vi "Client.vi"() -> ()   [LabVIEW 2020]
panel:
  in  "zone 6":bool
  in  "zone 5":bool
  in  "zone 4":bool
  in  "zone 3":bool
  in  "zone 2":bool
  in  "zone 1":bool
  in  "Alarm 6":bool
  in  "Alarm 5":bool
  in  "Alarm 4":bool
  in  "Alarm 3":bool
  in  "Alarm 2":bool
  in  "Alarm 1":bool
  in  "Bypass 6":bool
  in  "Bypass 5":bool
  in  "Bypass 4":bool
  in  "Bypass 3":bool
  in  "Bypass 2":bool
  in  "Bypass 1":bool
  in  "Temper 6":bool
  in  "Temper 5":bool
  in  "Temper 4":bool
  in  "Temper 3":bool
  in  "Temper 2":bool
  in  "Temper 1":bool
  # "1\n\n\n2\n\n\n3\n\n\n4\n\n\n5\n\n\n6"
  # "Bypass\nSwitches"
  # "Tamper\nSwitches"
  # "Alarm\nSwitches"
  # "Zone"
  # "Green = Normal\nRed = Alarm\nBlue = Bypass\nOrange = Tamper"
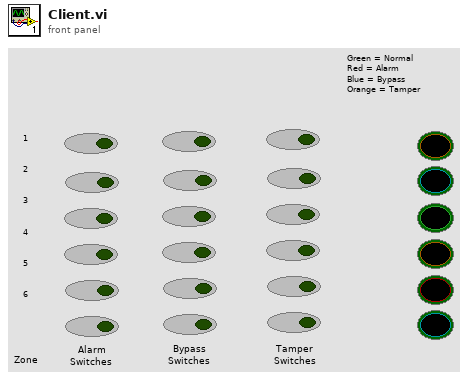
[diagram p1: front panel]
types:
  T1 = enum16{"Inti", "Wait", "zone 1", "zone 2", "zone 3", "zone 4", "zone 5", "zone 6"}
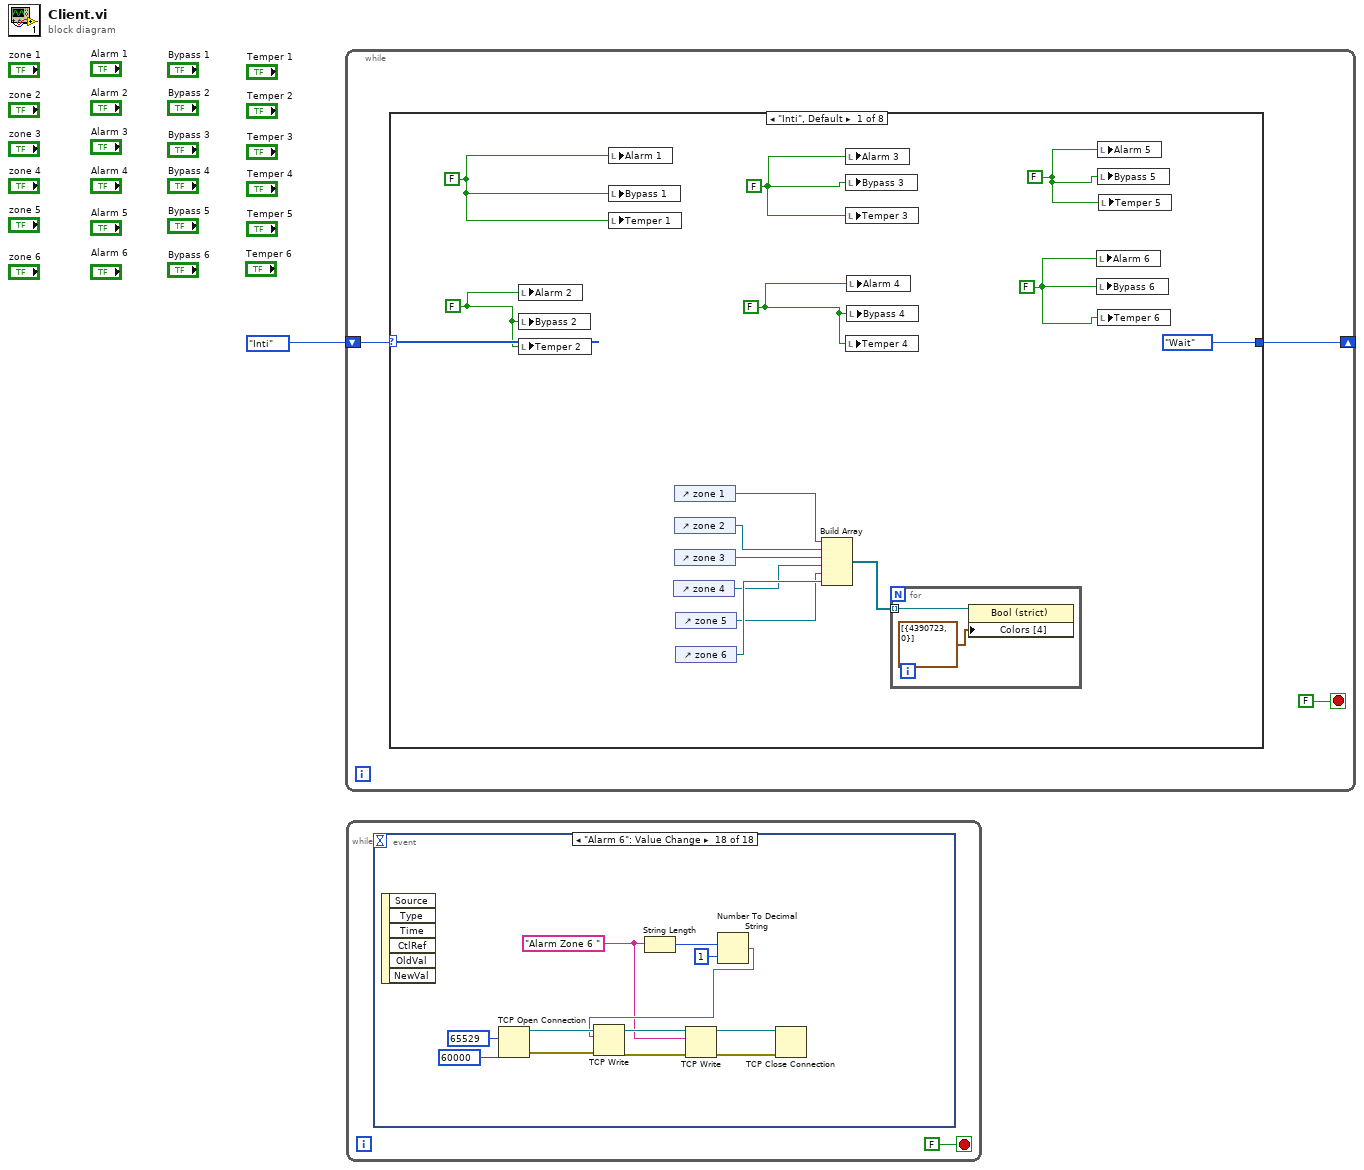
[diagram p0: block diagram]
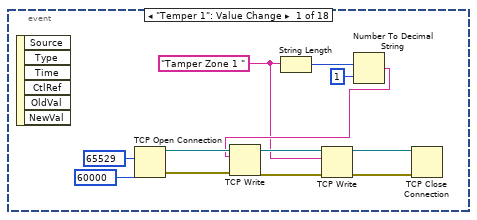
[diagram p2: hidden frame]
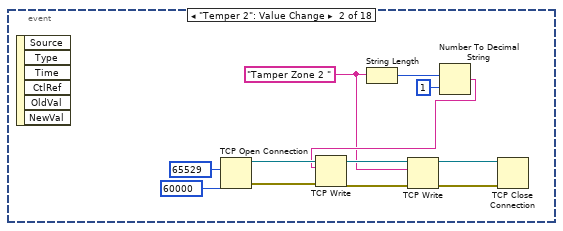
[diagram p3: hidden frame]
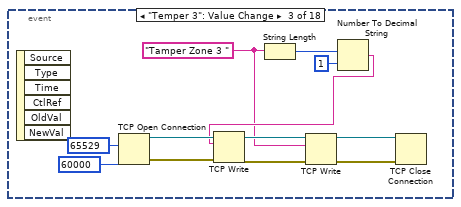
[diagram p4: hidden frame]
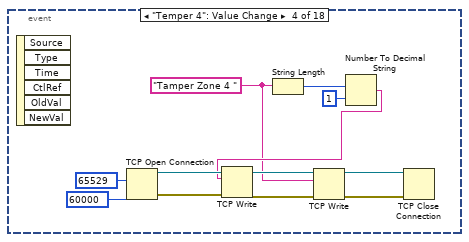
[diagram p5: hidden frame]
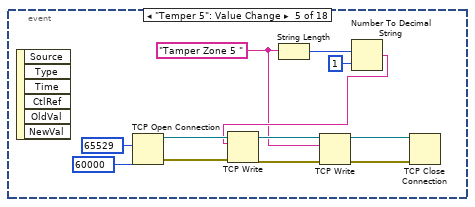
[diagram p6: hidden frame]
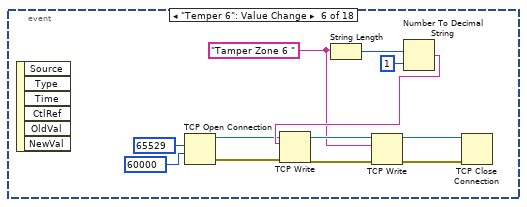
[diagram p7: hidden frame]
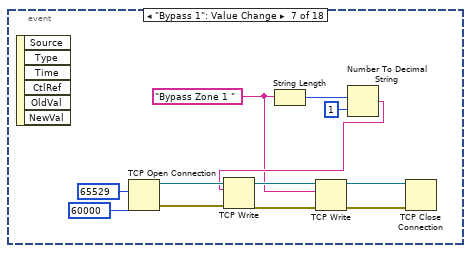
[diagram p8: hidden frame]
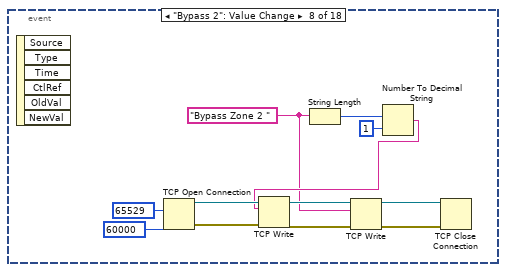
[diagram p9: hidden frame]
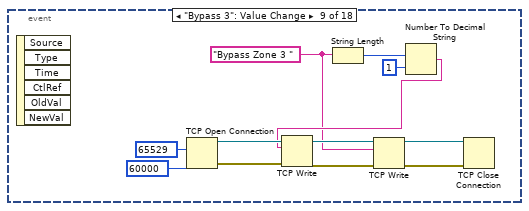
[diagram p10: hidden frame]
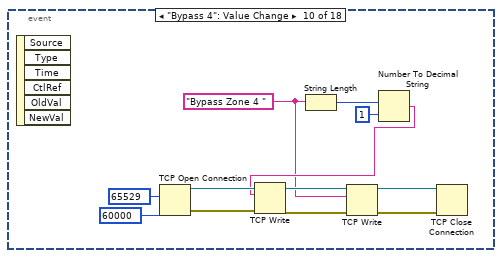
[diagram p11: hidden frame]
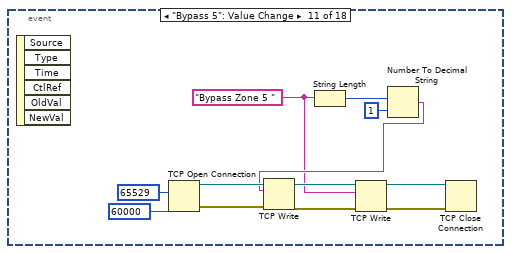
[diagram p12: hidden frame]
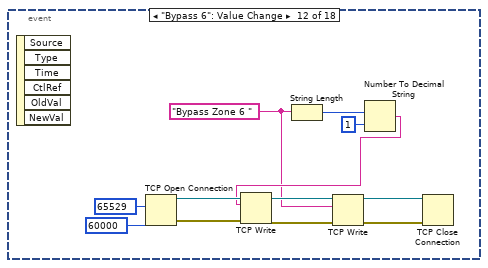
[diagram p13: hidden frame]
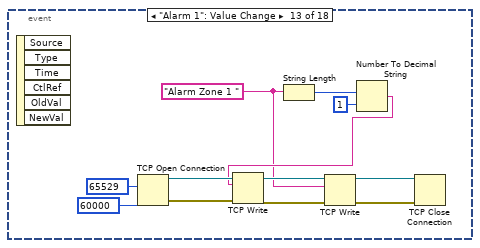
[diagram p14: hidden frame]
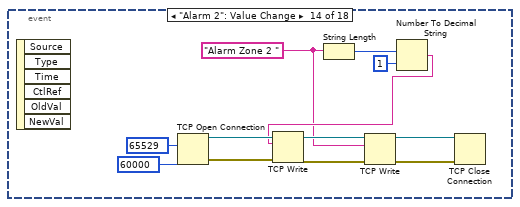
[diagram p15: hidden frame]
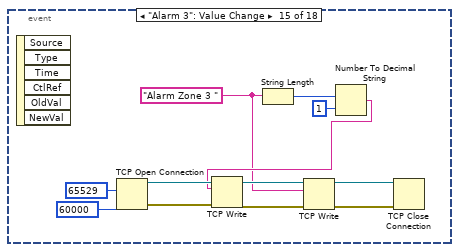
[diagram p16: hidden frame]
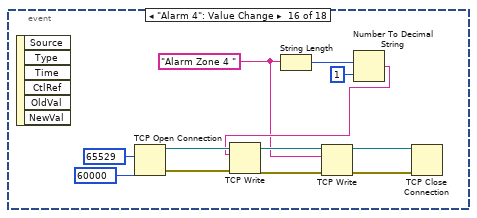
[diagram p17: hidden frame]
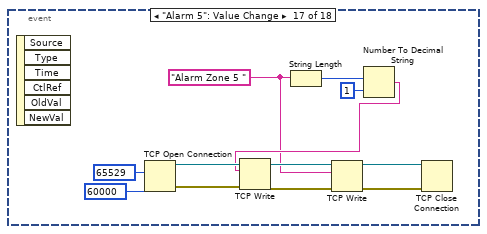
[diagram p18: hidden frame]
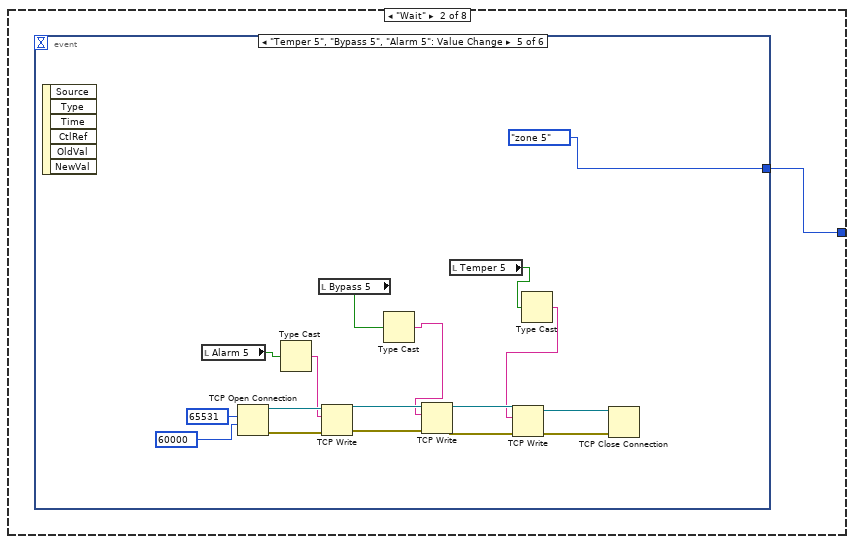
[diagram p19: hidden frame]
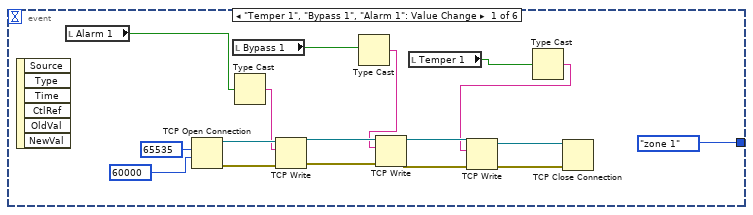
[diagram p20: hidden frame]
diagram:
  n1 = while {
    shift-right: [w2] -> _
    shift-left: T1."Inti" -> [w3]
    stop <- FALSE stop-if-true
    n2 = case shown="\"Inti\", Default" w3 {
      tunnel: [T1."Wait" w21 T1."Wait" T1."Wait" T1."Wait" T1."Wait" T1."Wait" T1."Wait"] -> w2
      frame "Inti", Default {
        w5 = FALSE
        w6 = FALSE
        w7 = FALSE
        w9 = FALSE
        w10 = FALSE
        w8 = FALSE
        n3 = local write "Alarm 2"(w10) -> ()
        n4 = local write "Bypass 2"(w10) -> ()
        n5 = local write "Temper 2"(w10) -> ()
        n6 = local write "Alarm 1"(w8) -> ()
        n7 = local write "Bypass 1"(w8) -> ()
        n8 = local write "Temper 1"(w8) -> ()
        n9 = control-ref of="zone 4"() -> (w15:refnum<vi>)
        n10 = control-ref of="zone 1"() -> (w12:refnum<vi>)
        n11 = control-ref of="zone 2"() -> (w13:refnum<vi>)
        n12 = control-ref of="zone 3"() -> (w14:refnum<vi>)
        n13 = control-ref of="zone 5"() -> (w16:refnum<vi>)
        n14 = control-ref of="zone 6"() -> (w17:refnum<vi>)
        n15 = Build Array "Build Array"(w12, w13, w14, w15, w16, w17) -> (w18:refnum<vi>[])
        n16 = local write "Alarm 3"(w9) -> ()
        n17 = local write "Bypass 3"(w9) -> ()
        n18 = local write "Temper 3"(w9) -> ()
        n19 = local write "Temper 4"(w7) -> ()
        n20 = local write "Alarm 4"(w7) -> ()
        n21 = local write "Bypass 4"(w7) -> ()
        n22 = for {
          tunnel: w18 -> [w19] mode=indexing
          n23 = property class="Bool (strict)"(reference=w19, "Colors [4]"=cluster{u32, u32}[] [{4390723, 0}] ("Couleurs [4]")) -> ()  [unwired: 1 in, 2 out]
        }
        n24 = local write "Alarm 6"(w5) -> ()
        n25 = local write "Bypass 6"(w5) -> ()
        n26 = local write "Alarm 5"(w6) -> ()
        n27 = local write "Bypass 5"(w6) -> ()
        n28 = local write "Temper 6"(w5) -> ()
        n29 = local write "Temper 5"(w6) -> ()
      }
      frame "Wait" {
        n30 = event shown="[4] \"Temper 5\", \"Bypass 5\", \"Alarm 5\": Value Change" {
          selector: _ -> [_ _ _ _ _ _]
          dyn-events: _ -> [_ _ _ _ _ _]
          timeout: _ -> [_ _ _ _ _ _]
          tunnel: [T1."zone 1" T1."zone 2" T1."zone 3" T1."zone 4" T1."zone 5" T1."zone 6"] -> w21
          event "Temper 1", "Bypass 1", "Alarm 1": Value Change {
            n31 = event-data() -> ()  [unwired: 1 in, 6 out]
            n32 = local read "Alarm 1"() -> (w35:bool)
            n33 = TCP Open Connection(remote port or service name=u16 65535, timeout ms (60000)=60000) -> (connection ID=w38:refnum<k5>, error out=w37:errorcluster)  [unwired: 3 in]
            n34 = local read "Bypass 1"() -> (w31:bool)
            n35 = Type Cast(x=w35) -> (*(type *) &x=w36:string)  [unwired: 1 in]
            n36 = TCP Write(connection ID=w38, data in=w36, error in (no error)=w37) -> (connection ID out=w29:refnum<k5>, error out=w28:errorcluster)  [unwired: 1 in, 1 out]
            n37 = Type Cast(x=w31) -> (*(type *) &x=w23:string)  [unwired: 1 in]
            n38 = TCP Write(connection ID=w29, data in=w23, error in (no error)=w28) -> (connection ID out=w27:refnum<k5>, error out=w26:errorcluster)  [unwired: 1 in, 1 out]
            n39 = local read "Temper 1"() -> (w30:bool)
            n40 = Type Cast(x=w30) -> (*(type *) &x=w22:string)  [unwired: 1 in]
            n41 = TCP Write(connection ID=w27, data in=w22, error in (no error)=w26) -> (connection ID out=w24:refnum<k5>, error out=w25:errorcluster)  [unwired: 1 in, 1 out]
            n42 = TCP Close Connection(connection ID=w24, error in (no error)=w25) -> ()  [unwired: 1 in, 2 out]
          }
          event "Temper 2", "Bypass 2", "Alarm 2": Value Change {
            n43 = event-data() -> ()  [unwired: 1 in, 6 out]
            n44 = local read "Alarm 2"() -> (w39:bool)
            n45 = TCP Open Connection(remote port or service name=u16 65534, timeout ms (60000)=60000) -> (connection ID=w54:refnum<k5>, error out=w53:errorcluster)  [unwired: 3 in]
            n46 = Type Cast(x=w39) -> (*(type *) &x=w52:string)  [unwired: 1 in]
            n47 = local read "Bypass 2"() -> (w40:bool)
            n48 = TCP Write(connection ID=w54, data in=w52, error in (no error)=w53) -> (connection ID out=w49:refnum<k5>, error out=w48:errorcluster)  [unwired: 1 in, 1 out]
            n49 = Type Cast(x=w40) -> (*(type *) &x=w42:string)  [unwired: 1 in]
            n50 = TCP Write(connection ID=w49, data in=w42, error in (no error)=w48) -> (connection ID out=w47:refnum<k5>, error out=w46:errorcluster)  [unwired: 1 in, 1 out]
            n51 = local read "Temper 2"() -> (w41:bool)
            n52 = Type Cast(x=w41) -> (*(type *) &x=w43:string)  [unwired: 1 in]
            n53 = TCP Write(connection ID=w47, data in=w43, error in (no error)=w46) -> (connection ID out=w44:refnum<k5>, error out=w45:errorcluster)  [unwired: 1 in, 1 out]
            n54 = TCP Close Connection(connection ID=w44, error in (no error)=w45) -> ()  [unwired: 1 in, 2 out]
          }
          event "Temper 3", "Bypass 3", "Alarm 3": Value Change {
            n55 = event-data() -> ()  [unwired: 1 in, 6 out]
            n56 = local read "Alarm 3"() -> (w56:bool)
            n57 = TCP Open Connection(remote port or service name=u16 65533, timeout ms (60000)=60000) -> (connection ID=w71:refnum<k5>, error out=w70:errorcluster)  [unwired: 3 in]
            n58 = Type Cast(x=w56) -> (*(type *) &x=w69:string)  [unwired: 1 in]
            n59 = local read "Bypass 3"() -> (w58:bool)
            n60 = TCP Write(connection ID=w71, data in=w69, error in (no error)=w70) -> (connection ID out=w66:refnum<k5>, error out=w65:errorcluster)  [unwired: 1 in, 1 out]
            n61 = Type Cast(x=w58) -> (*(type *) &x=w59:string)  [unwired: 1 in]
            n62 = TCP Write(connection ID=w66, data in=w59, error in (no error)=w65) -> (connection ID out=w64:refnum<k5>, error out=w63:errorcluster)  [unwired: 1 in, 1 out]
            n63 = local read "Temper 3"() -> (w57:bool)
            n64 = Type Cast(x=w57) -> (*(type *) &x=w60:string)  [unwired: 1 in]
            n65 = TCP Write(connection ID=w64, data in=w60, error in (no error)=w63) -> (connection ID out=w61:refnum<k5>, error out=w62:errorcluster)  [unwired: 1 in, 1 out]
            n66 = TCP Close Connection(connection ID=w61, error in (no error)=w62) -> ()  [unwired: 1 in, 2 out]
          }
          event "Temper 4", "Bypass 4", "Alarm 4": Value Change {
            n67 = event-data() -> ()  [unwired: 1 in, 6 out]
            n68 = local read "Alarm 4"() -> (w75:bool)
            n69 = TCP Open Connection(remote port or service name=u16 65532, timeout ms (60000)=60000) -> (connection ID=w88:refnum<k5>, error out=w87:errorcluster)  [unwired: 3 in]
            n70 = Type Cast(x=w75) -> (*(type *) &x=w86:string)  [unwired: 1 in]
            n71 = TCP Write(connection ID=w88, data in=w86, error in (no error)=w87) -> (connection ID out=w83:refnum<k5>, error out=w82:errorcluster)  [unwired: 1 in, 1 out]
            n72 = local read "Bypass 4"() -> (w74:bool)
            n73 = Type Cast(x=w74) -> (*(type *) &x=w76:string)  [unwired: 1 in]
            n74 = TCP Write(connection ID=w83, data in=w76, error in (no error)=w82) -> (connection ID out=w81:refnum<k5>, error out=w80:errorcluster)  [unwired: 1 in, 1 out]
            n75 = local read "Temper 4"() -> (w73:bool)
            n76 = Type Cast(x=w73) -> (*(type *) &x=w77:string)  [unwired: 1 in]
            n77 = TCP Write(connection ID=w81, data in=w77, error in (no error)=w80) -> (connection ID out=w78:refnum<k5>, error out=w79:errorcluster)  [unwired: 1 in, 1 out]
            n78 = TCP Close Connection(connection ID=w78, error in (no error)=w79) -> ()  [unwired: 1 in, 2 out]
          }
          event "Temper 5", "Bypass 5", "Alarm 5": Value Change {
            n79 = event-data() -> ()  [unwired: 1 in, 6 out]
            n80 = local read "Alarm 5"() -> (w92:bool)
            n81 = TCP Open Connection(remote port or service name=u16 65531, timeout ms (60000)=60000) -> (connection ID=w105:refnum<k5>, error out=w104:errorcluster)  [unwired: 3 in]
            n82 = Type Cast(x=w92) -> (*(type *) &x=w103:string)  [unwired: 1 in]
            n83 = local read "Bypass 5"() -> (w91:bool)
            n84 = TCP Write(connection ID=w105, data in=w103, error in (no error)=w104) -> (connection ID out=w100:refnum<k5>, error out=w99:errorcluster)  [unwired: 1 in, 1 out]
            n85 = Type Cast(x=w91) -> (*(type *) &x=w93:string)  [unwired: 1 in]
            n86 = TCP Write(connection ID=w100, data in=w93, error in (no error)=w99) -> (connection ID out=w98:refnum<k5>, error out=w97:errorcluster)  [unwired: 1 in, 1 out]
            n87 = local read "Temper 5"() -> (w90:bool)
            n88 = Type Cast(x=w90) -> (*(type *) &x=w94:string)  [unwired: 1 in]
            n89 = TCP Write(connection ID=w98, data in=w94, error in (no error)=w97) -> (connection ID out=w95:refnum<k5>, error out=w96:errorcluster)  [unwired: 1 in, 1 out]
            n90 = TCP Close Connection(connection ID=w95, error in (no error)=w96) -> ()  [unwired: 1 in, 2 out]
          }
          event "Temper 6", "Bypass 6", "Alarm 6": Value Change {
            n91 = event-data() -> ()  [unwired: 1 in, 6 out]
            n92 = local read "Alarm 6"() -> (w109:bool)
            n93 = TCP Open Connection(remote port or service name=u16 65530, timeout ms (60000)=60000) -> (connection ID=w123:refnum<k5>, error out=w122:errorcluster)  [unwired: 3 in]
            n94 = Type Cast(x=w109) -> (*(type *) &x=w121:string)  [unwired: 1 in]
            n95 = TCP Write(connection ID=w123, data in=w121, error in (no error)=w122) -> (connection ID out=w118:refnum<k5>, error out=w117:errorcluster)  [unwired: 1 in, 1 out]
            n96 = local read "Bypass 6"() -> (w108:bool)
            n97 = Type Cast(x=w108) -> (*(type *) &x=w111:string)  [unwired: 1 in]
            n98 = TCP Write(connection ID=w118, data in=w111, error in (no error)=w117) -> (connection ID out=w116:refnum<k5>, error out=w115:errorcluster)  [unwired: 1 in, 1 out]
            n99 = local read "Temper 6"() -> (w107:bool)
            n100 = Type Cast(x=w107) -> (*(type *) &x=w112:string)  [unwired: 1 in]
            n101 = TCP Write(connection ID=w116, data in=w112, error in (no error)=w115) -> (connection ID out=w113:refnum<k5>, error out=w114:errorcluster)  [unwired: 1 in, 1 out]
            n102 = TCP Close Connection(connection ID=w113, error in (no error)=w114) -> ()  [unwired: 1 in, 2 out]
          }
        }
      }
      frame "zone 1" {
        n103 = local read "Temper 1"() -> (w126:bool)
        n104 = local read "Bypass 1"() -> (w125:bool)
        n105 = local read "Alarm 1"() -> (w124:bool)
        n106 = case shown="False" w126 {
          tunnel: w125 -> [w129 _]
          tunnel: w124 -> [w128 _]
          frame False {
            n107 = case shown="False" w129 {
              tunnel: w128 -> [w130 _]
              frame False {
                n108 = case shown="True" w130 {
                  frame False {
                    n109 = property on="zone 1" class="Bool (strict)"("Colors [4]"=cluster{u32, i32}[] [{6618880, 0}]) -> ()  [unwired: 2 in, 2 out]
                  }
                  frame True {
                    n110 = property on="zone 1" class="Bool (strict)"("Colors [4]"=cluster{u32, i32}[] [{16711680, 0}]) -> ()  [unwired: 2 in, 2 out]
                  }
                }
              }
              frame True {
                n111 = property on="zone 1" class="Bool (strict)"("Colors [4]"=cluster{u32, i32}[] [{59391, 0}]) -> ()  [unwired: 2 in, 2 out]
              }
            }
          }
          frame True {
            n112 = property on="zone 1" class="Bool (strict)"("Colors [4]"=cluster{u32, i32}[] [{16748288, 0}]) -> ()  [unwired: 2 in, 2 out]
          }
        }
      }
      frame "zone 2" {
        n113 = local read "Temper 2"() -> (w135:bool)
        n114 = local read "Alarm 2"() -> (w137:bool)
        n115 = local read "Bypass 2"() -> (w136:bool)
        n116 = case shown="False" w135 {
          tunnel: w136 -> [w140 _]
          tunnel: w137 -> [w139 _]
          frame False {
            n117 = case shown="False" w140 {
              tunnel: w139 -> [w141 _]
              frame False {
                n118 = case shown="True" w141 {
                  frame False {
                    n119 = property on="zone 2" class="Bool (strict)"("Colors [4]"=cluster{u32, i32}[] [{6618880, 0}]) -> ()  [unwired: 2 in, 2 out]
                  }
                  frame True {
                    n120 = property on="zone 2" class="Bool (strict)"("Colors [4]"=cluster{u32, i32}[] [{16711680, 0}]) -> ()  [unwired: 2 in, 2 out]
                  }
                }
              }
              frame True {
                n121 = property on="zone 2" class="Bool (strict)"("Colors [4]"=cluster{u32, i32}[] [{59391, 0}]) -> ()  [unwired: 2 in, 2 out]
              }
            }
          }
          frame True {
            n122 = property on="zone 2" class="Bool (strict)"("Colors [4]"=cluster{u32, i32}[] [{16748288, 0}]) -> ()  [unwired: 2 in, 2 out]
          }
        }
      }
      frame "zone 3" {
        n123 = local read "Bypass 3"() -> (w147:bool)
        n124 = local read "Alarm 3"() -> (w148:bool)
        n125 = local read "Temper 3"() -> (w146:bool)
        n126 = case shown="False" w146 {
          tunnel: w147 -> [w151 _]
          tunnel: w148 -> [w150 _]
          frame False {
            n127 = case shown="False" w151 {
              tunnel: w150 -> [w152 _]
              frame False {
                n128 = case shown="False" w152 {
                  frame False {
                    n129 = property on="zone 3" class="Bool (strict)"("Colors [4]"=cluster{u32, i32}[] [{6618880, 0}]) -> ()  [unwired: 2 in, 2 out]
                  }
                  frame True {
                    n130 = property on="zone 3" class="Bool (strict)"("Colors [4]"=cluster{u32, i32}[] [{16711680, 0}]) -> ()  [unwired: 2 in, 2 out]
                  }
                }
              }
              frame True {
                n131 = property on="zone 3" class="Bool (strict)"("Colors [4]"=cluster{u32, i32}[] [{59391, 0}]) -> ()  [unwired: 2 in, 2 out]
              }
            }
          }
          frame True {
            n132 = property on="zone 3" class="Bool (strict)"("Colors [4]"=cluster{u32, i32}[] [{16748288, 0}]) -> ()  [unwired: 2 in, 2 out]
          }
        }
      }
      frame "zone 4" {
        n133 = local read "Temper 4"() -> (w159:bool)
        n134 = local read "Bypass 4"() -> (w158:bool)
        n135 = local read "Alarm 4"() -> (w157:bool)
        n136 = case shown="True" w159 {
          tunnel: w158 -> [w162 _]
          tunnel: w157 -> [w161 _]
          frame False {
            n137 = case shown="True" w162 {
              tunnel: w161 -> [w163 _]
              frame False {
                n138 = case shown="True" w163 {
                  frame False {
                    n139 = property on="zone 4" class="Bool (strict)"("Colors [4]"=cluster{u32, i32}[] [{6618880, 0}]) -> ()  [unwired: 2 in, 2 out]
                  }
                  frame True {
                    n140 = property on="zone 4" class="Bool (strict)"("Colors [4]"=cluster{u32, i32}[] [{16711680, 0}]) -> ()  [unwired: 2 in, 2 out]
                  }
                }
              }
              frame True {
                n141 = property on="zone 4" class="Bool (strict)"("Colors [4]"=cluster{u32, i32}[] [{59391, 0}]) -> ()  [unwired: 2 in, 2 out]
              }
            }
          }
          frame True {
            n142 = property on="zone 4" class="Bool (strict)"("Colors [4]"=cluster{u32, i32}[] [{16748288, 0}]) -> ()  [unwired: 2 in, 2 out]
          }
        }
      }
      frame "zone 5" {
        n143 = local read "Temper 5"() -> (w168:bool)
        n144 = local read "Alarm 5"() -> (w170:bool)
        n145 = local read "Bypass 5"() -> (w169:bool)
        n146 = case shown="True" w168 {
          tunnel: w169 -> [w173 _]
          tunnel: w170 -> [w172 _]
          frame False {
            n147 = case shown="True" w173 {
              tunnel: w172 -> [w174 _]
              frame False {
                n148 = case shown="True" w174 {
                  frame False {
                    n149 = property on="zone 5" class="Bool (strict)"("Colors [4]"=cluster{u32, i32}[] [{6618880, 0}]) -> ()  [unwired: 2 in, 2 out]
                  }
                  frame True {
                    n150 = property on="zone 5" class="Bool (strict)"("Colors [4]"=cluster{u32, i32}[] [{16711680, 0}]) -> ()  [unwired: 2 in, 2 out]
                  }
                }
              }
              frame True {
                n151 = property on="zone 5" class="Bool (strict)"("Colors [4]"=cluster{u32, i32}[] [{59391, 0}]) -> ()  [unwired: 2 in, 2 out]
              }
            }
          }
          frame True {
            n152 = property on="zone 5" class="Bool (strict)"("Colors [4]"=cluster{u32, i32}[] [{16748288, 0}]) -> ()  [unwired: 2 in, 2 out]
          }
        }
      }
      frame "zone 6" {
        n153 = local read "Temper 6"() -> (w179:bool)
        n154 = local read "Bypass 6"() -> (w180:bool)
        n155 = local read "Alarm 6"() -> (w181:bool)
        n156 = case shown="True" w179 {
          tunnel: w180 -> [w184 _]
          tunnel: w181 -> [w183 _]
          frame False {
            n157 = case shown="True" w184 {
              tunnel: w183 -> [w185 _]
              frame False {
                n158 = case shown="True" w185 {
                  frame False {
                    n159 = property on="zone 6" class="Bool (strict)"("Colors [4]"=cluster{u32, i32}[] [{6618880, 0}]) -> ()  [unwired: 2 in, 2 out]
                  }
                  frame True {
                    n160 = property on="zone 6" class="Bool (strict)"("Colors [4]"=cluster{u32, i32}[] [{16711680, 0}]) -> ()  [unwired: 2 in, 2 out]
                  }
                }
              }
              frame True {
                n161 = property on="zone 6" class="Bool (strict)"("Colors [4]"=cluster{u32, i32}[] [{59391, 0}]) -> ()  [unwired: 2 in, 2 out]
              }
            }
          }
          frame True {
            n162 = property on="zone 6" class="Bool (strict)"("Colors [4]"=cluster{u32, i32}[] [{16748288, 0}]) -> ()  [unwired: 2 in, 2 out]
          }
        }
      }
    }
  }
  n163 = while {
    stop <- FALSE stop-if-true
    n164 = event shown="[17] \"Alarm 6\": Value Change" {
      selector: _ -> [_ _ _ _ _ _ _ _ _ _ _ _ _ _ _ _ _ _]
      dyn-events: _ -> [_ _ _ _ _ _ _ _ _ _ _ _ _ _ _ _ _ _]
      timeout: _ -> [_ _ _ _ _ _ _ _ _ _ _ _ _ _ _ _ _ _]
      event "Temper 1": Value Change {
        w191 = "Tamper Zone 1 "
        n165 = event-data() -> ()  [unwired: 1 in, 6 out]
        n166 = TCP Open Connection(remote port or service name=u16 65529, timeout ms (60000)=60000) -> (connection ID=w202:refnum<k5>, error out=w201:errorcluster)  [unwired: 3 in]
        n167 = String Length(string=w191) -> (length=w198:i32)
        n168 = Number To Decimal String(number=w198, width (-)=i16 1) -> (decimal integer string=w196:string)
        n169 = TCP Write(connection ID=w202, data in=w196, error in (no error)=w201) -> (connection ID out=w195:refnum<k5>, error out=w194:errorcluster)  [unwired: 1 in, 1 out]
        n170 = TCP Write(connection ID=w195, data in=w191, error in (no error)=w194) -> (connection ID out=w193:refnum<k5>, error out=w192:errorcluster)  [unwired: 1 in, 1 out]
        n171 = TCP Close Connection(connection ID=w193, error in (no error)=w192) -> ()  [unwired: 1 in, 2 out]
      }
      event "Temper 2": Value Change {
        w203 = "Tamper Zone 2 "
        n172 = event-data() -> ()  [unwired: 1 in, 6 out]
        n173 = TCP Open Connection(remote port or service name=u16 65529, timeout ms (60000)=60000) -> (connection ID=w214:refnum<k5>, error out=w213:errorcluster)  [unwired: 3 in]
        n174 = String Length(string=w203) -> (length=w210:i32)
        n175 = Number To Decimal String(number=w210, width (-)=i16 1) -> (decimal integer string=w208:string)
        n176 = TCP Write(connection ID=w214, data in=w208, error in (no error)=w213) -> (connection ID out=w207:refnum<k5>, error out=w206:errorcluster)  [unwired: 1 in, 1 out]
        n177 = TCP Write(connection ID=w207, data in=w203, error in (no error)=w206) -> (connection ID out=w205:refnum<k5>, error out=w204:errorcluster)  [unwired: 1 in, 1 out]
        n178 = TCP Close Connection(connection ID=w205, error in (no error)=w204) -> ()  [unwired: 1 in, 2 out]
      }
      event "Temper 3": Value Change {
        w215 = "Tamper Zone 3 "
        n179 = event-data() -> ()  [unwired: 1 in, 6 out]
        n180 = TCP Open Connection(remote port or service name=u16 65529, timeout ms (60000)=60000) -> (connection ID=w226:refnum<k5>, error out=w225:errorcluster)  [unwired: 3 in]
        n181 = String Length(string=w215) -> (length=w222:i32)
        n182 = Number To Decimal String(number=w222, width (-)=i16 1) -> (decimal integer string=w220:string)
        n183 = TCP Write(connection ID=w226, data in=w220, error in (no error)=w225) -> (connection ID out=w219:refnum<k5>, error out=w218:errorcluster)  [unwired: 1 in, 1 out]
        n184 = TCP Write(connection ID=w219, data in=w215, error in (no error)=w218) -> (connection ID out=w217:refnum<k5>, error out=w216:errorcluster)  [unwired: 1 in, 1 out]
        n185 = TCP Close Connection(connection ID=w217, error in (no error)=w216) -> ()  [unwired: 1 in, 2 out]
      }
      event "Temper 4": Value Change {
        w227 = "Tamper Zone 4 "
        n186 = event-data() -> ()  [unwired: 1 in, 6 out]
        n187 = TCP Open Connection(remote port or service name=u16 65529, timeout ms (60000)=60000) -> (connection ID=w238:refnum<k5>, error out=w237:errorcluster)  [unwired: 3 in]
        n188 = String Length(string=w227) -> (length=w234:i32)
        n189 = Number To Decimal String(number=w234, width (-)=i16 1) -> (decimal integer string=w232:string)
        n190 = TCP Write(connection ID=w238, data in=w232, error in (no error)=w237) -> (connection ID out=w231:refnum<k5>, error out=w230:errorcluster)  [unwired: 1 in, 1 out]
        n191 = TCP Write(connection ID=w231, data in=w227, error in (no error)=w230) -> (connection ID out=w229:refnum<k5>, error out=w228:errorcluster)  [unwired: 1 in, 1 out]
        n192 = TCP Close Connection(connection ID=w229, error in (no error)=w228) -> ()  [unwired: 1 in, 2 out]
      }
      event "Temper 5": Value Change {
        w239 = "Tamper Zone 5 "
        n193 = event-data() -> ()  [unwired: 1 in, 6 out]
        n194 = TCP Open Connection(remote port or service name=u16 65529, timeout ms (60000)=60000) -> (connection ID=w250:refnum<k5>, error out=w249:errorcluster)  [unwired: 3 in]
        n195 = String Length(string=w239) -> (length=w246:i32)
        n196 = Number To Decimal String(number=w246, width (-)=i16 1) -> (decimal integer string=w244:string)
        n197 = TCP Write(connection ID=w250, data in=w244, error in (no error)=w249) -> (connection ID out=w243:refnum<k5>, error out=w242:errorcluster)  [unwired: 1 in, 1 out]
        n198 = TCP Write(connection ID=w243, data in=w239, error in (no error)=w242) -> (connection ID out=w241:refnum<k5>, error out=w240:errorcluster)  [unwired: 1 in, 1 out]
        n199 = TCP Close Connection(connection ID=w241, error in (no error)=w240) -> ()  [unwired: 1 in, 2 out]
      }
      event "Temper 6": Value Change {
        w252 = "Tamper Zone 6 "
        n200 = event-data() -> ()  [unwired: 1 in, 6 out]
        n201 = TCP Open Connection(remote port or service name=u16 65529, timeout ms (60000)=60000) -> (connection ID=w255:refnum<k5>, error out=w256:errorcluster)  [unwired: 3 in]
        n202 = String Length(string=w252) -> (length=w257:i32)
        n203 = Number To Decimal String(number=w257, width (-)=i16 1) -> (decimal integer string=w258:string)
        n204 = TCP Write(connection ID=w255, data in=w258, error in (no error)=w256) -> (connection ID out=w259:refnum<k5>, error out=w260:errorcluster)  [unwired: 1 in, 1 out]
        n205 = TCP Write(connection ID=w259, data in=w252, error in (no error)=w260) -> (connection ID out=w261:refnum<k5>, error out=w262:errorcluster)  [unwired: 1 in, 1 out]
        n206 = TCP Close Connection(connection ID=w261, error in (no error)=w262) -> ()  [unwired: 1 in, 2 out]
      }
      event "Bypass 1": Value Change {
        w263 = "Bypass Zone 1 "
        n207 = event-data() -> ()  [unwired: 1 in, 6 out]
        n208 = TCP Open Connection(remote port or service name=u16 65529, timeout ms (60000)=60000) -> (connection ID=w274:refnum<k5>, error out=w273:errorcluster)  [unwired: 3 in]
        n209 = String Length(string=w263) -> (length=w270:i32)
        n210 = Number To Decimal String(number=w270, width (-)=i16 1) -> (decimal integer string=w268:string)
        n211 = TCP Write(connection ID=w274, data in=w268, error in (no error)=w273) -> (connection ID out=w267:refnum<k5>, error out=w266:errorcluster)  [unwired: 1 in, 1 out]
        n212 = TCP Write(connection ID=w267, data in=w263, error in (no error)=w266) -> (connection ID out=w265:refnum<k5>, error out=w264:errorcluster)  [unwired: 1 in, 1 out]
        n213 = TCP Close Connection(connection ID=w265, error in (no error)=w264) -> ()  [unwired: 1 in, 2 out]
      }
      event "Bypass 2": Value Change {
        w275 = "Bypass Zone 2 "
        n214 = event-data() -> ()  [unwired: 1 in, 6 out]
        n215 = TCP Open Connection(remote port or service name=u16 65529, timeout ms (60000)=60000) -> (connection ID=w286:refnum<k5>, error out=w285:errorcluster)  [unwired: 3 in]
        n216 = String Length(string=w275) -> (length=w282:i32)
        n217 = Number To Decimal String(number=w282, width (-)=i16 1) -> (decimal integer string=w280:string)
        n218 = TCP Write(connection ID=w286, data in=w280, error in (no error)=w285) -> (connection ID out=w279:refnum<k5>, error out=w278:errorcluster)  [unwired: 1 in, 1 out]
        n219 = TCP Write(connection ID=w279, data in=w275, error in (no error)=w278) -> (connection ID out=w277:refnum<k5>, error out=w276:errorcluster)  [unwired: 1 in, 1 out]
        n220 = TCP Close Connection(connection ID=w277, error in (no error)=w276) -> ()  [unwired: 1 in, 2 out]
      }
      event "Bypass 3": Value Change {
        w287 = "Bypass Zone 3 "
        n221 = event-data() -> ()  [unwired: 1 in, 6 out]
        n222 = TCP Open Connection(remote port or service name=u16 65529, timeout ms (60000)=60000) -> (connection ID=w298:refnum<k5>, error out=w297:errorcluster)  [unwired: 3 in]
        n223 = String Length(string=w287) -> (length=w294:i32)
        n224 = Number To Decimal String(number=w294, width (-)=i16 1) -> (decimal integer string=w292:string)
        n225 = TCP Write(connection ID=w298, data in=w292, error in (no error)=w297) -> (connection ID out=w291:refnum<k5>, error out=w290:errorcluster)  [unwired: 1 in, 1 out]
        n226 = TCP Write(connection ID=w291, data in=w287, error in (no error)=w290) -> (connection ID out=w289:refnum<k5>, error out=w288:errorcluster)  [unwired: 1 in, 1 out]
        n227 = TCP Close Connection(connection ID=w289, error in (no error)=w288) -> ()  [unwired: 1 in, 2 out]
      }
      event "Bypass 4": Value Change {
        w299 = "Bypass Zone 4 "
        n228 = event-data() -> ()  [unwired: 1 in, 6 out]
        n229 = TCP Open Connection(remote port or service name=u16 65529, timeout ms (60000)=60000) -> (connection ID=w310:refnum<k5>, error out=w309:errorcluster)  [unwired: 3 in]
        n230 = String Length(string=w299) -> (length=w306:i32)
        n231 = Number To Decimal String(number=w306, width (-)=i16 1) -> (decimal integer string=w304:string)
        n232 = TCP Write(connection ID=w310, data in=w304, error in (no error)=w309) -> (connection ID out=w303:refnum<k5>, error out=w302:errorcluster)  [unwired: 1 in, 1 out]
        n233 = TCP Write(connection ID=w303, data in=w299, error in (no error)=w302) -> (connection ID out=w301:refnum<k5>, error out=w300:errorcluster)  [unwired: 1 in, 1 out]
        n234 = TCP Close Connection(connection ID=w301, error in (no error)=w300) -> ()  [unwired: 1 in, 2 out]
      }
      event "Bypass 5": Value Change {
        w311 = "Bypass Zone 5 "
        n235 = event-data() -> ()  [unwired: 1 in, 6 out]
        n236 = TCP Open Connection(remote port or service name=u16 65529, timeout ms (60000)=60000) -> (connection ID=w322:refnum<k5>, error out=w321:errorcluster)  [unwired: 3 in]
        n237 = String Length(string=w311) -> (length=w318:i32)
        n238 = Number To Decimal String(number=w318, width (-)=i16 1) -> (decimal integer string=w316:string)
        n239 = TCP Write(connection ID=w322, data in=w316, error in (no error)=w321) -> (connection ID out=w315:refnum<k5>, error out=w314:errorcluster)  [unwired: 1 in, 1 out]
        n240 = TCP Write(connection ID=w315, data in=w311, error in (no error)=w314) -> (connection ID out=w313:refnum<k5>, error out=w312:errorcluster)  [unwired: 1 in, 1 out]
        n241 = TCP Close Connection(connection ID=w313, error in (no error)=w312) -> ()  [unwired: 1 in, 2 out]
      }
      event "Bypass 6": Value Change {
        w323 = "Bypass Zone 6 "
        n242 = event-data() -> ()  [unwired: 1 in, 6 out]
        n243 = TCP Open Connection(remote port or service name=u16 65529, timeout ms (60000)=60000) -> (connection ID=w334:refnum<k5>, error out=w333:errorcluster)  [unwired: 3 in]
        n244 = String Length(string=w323) -> (length=w330:i32)
        n245 = Number To Decimal String(number=w330, width (-)=i16 1) -> (decimal integer string=w328:string)
        n246 = TCP Write(connection ID=w334, data in=w328, error in (no error)=w333) -> (connection ID out=w327:refnum<k5>, error out=w326:errorcluster)  [unwired: 1 in, 1 out]
        n247 = TCP Write(connection ID=w327, data in=w323, error in (no error)=w326) -> (connection ID out=w325:refnum<k5>, error out=w324:errorcluster)  [unwired: 1 in, 1 out]
        n248 = TCP Close Connection(connection ID=w325, error in (no error)=w324) -> ()  [unwired: 1 in, 2 out]
      }
      event "Alarm 1": Value Change {
        w335 = "Alarm Zone 1 "
        n249 = event-data() -> ()  [unwired: 1 in, 6 out]
        n250 = TCP Open Connection(remote port or service name=u16 65529, timeout ms (60000)=60000) -> (connection ID=w346:refnum<k5>, error out=w345:errorcluster)  [unwired: 3 in]
        n251 = String Length(string=w335) -> (length=w342:i32)
        n252 = Number To Decimal String(number=w342, width (-)=i16 1) -> (decimal integer string=w340:string)
        n253 = TCP Write(connection ID=w346, data in=w340, error in (no error)=w345) -> (connection ID out=w339:refnum<k5>, error out=w338:errorcluster)  [unwired: 1 in, 1 out]
        n254 = TCP Write(connection ID=w339, data in=w335, error in (no error)=w338) -> (connection ID out=w337:refnum<k5>, error out=w336:errorcluster)  [unwired: 1 in, 1 out]
        n255 = TCP Close Connection(connection ID=w337, error in (no error)=w336) -> ()  [unwired: 1 in, 2 out]
      }
      event "Alarm 2": Value Change {
        w347 = "Alarm Zone 2 "
        n256 = event-data() -> ()  [unwired: 1 in, 6 out]
        n257 = TCP Open Connection(remote port or service name=u16 65529, timeout ms (60000)=60000) -> (connection ID=w358:refnum<k5>, error out=w357:errorcluster)  [unwired: 3 in]
        n258 = String Length(string=w347) -> (length=w354:i32)
        n259 = Number To Decimal String(number=w354, width (-)=i16 1) -> (decimal integer string=w352:string)
        n260 = TCP Write(connection ID=w358, data in=w352, error in (no error)=w357) -> (connection ID out=w351:refnum<k5>, error out=w350:errorcluster)  [unwired: 1 in, 1 out]
        n261 = TCP Write(connection ID=w351, data in=w347, error in (no error)=w350) -> (connection ID out=w349:refnum<k5>, error out=w348:errorcluster)  [unwired: 1 in, 1 out]
        n262 = TCP Close Connection(connection ID=w349, error in (no error)=w348) -> ()  [unwired: 1 in, 2 out]
      }
      event "Alarm 3": Value Change {
        w359 = "Alarm Zone 3 "
        n263 = event-data() -> ()  [unwired: 1 in, 6 out]
        n264 = TCP Open Connection(remote port or service name=u16 65529, timeout ms (60000)=60000) -> (connection ID=w370:refnum<k5>, error out=w369:errorcluster)  [unwired: 3 in]
        n265 = String Length(string=w359) -> (length=w366:i32)
        n266 = Number To Decimal String(number=w366, width (-)=i16 1) -> (decimal integer string=w364:string)
        n267 = TCP Write(connection ID=w370, data in=w364, error in (no error)=w369) -> (connection ID out=w363:refnum<k5>, error out=w362:errorcluster)  [unwired: 1 in, 1 out]
        n268 = TCP Write(connection ID=w363, data in=w359, error in (no error)=w362) -> (connection ID out=w361:refnum<k5>, error out=w360:errorcluster)  [unwired: 1 in, 1 out]
        n269 = TCP Close Connection(connection ID=w361, error in (no error)=w360) -> ()  [unwired: 1 in, 2 out]
      }
      event "Alarm 4": Value Change {
        w371 = "Alarm Zone 4 "
        n270 = event-data() -> ()  [unwired: 1 in, 6 out]
        n271 = TCP Open Connection(remote port or service name=u16 65529, timeout ms (60000)=60000) -> (connection ID=w382:refnum<k5>, error out=w381:errorcluster)  [unwired: 3 in]
        n272 = String Length(string=w371) -> (length=w378:i32)
        n273 = Number To Decimal String(number=w378, width (-)=i16 1) -> (decimal integer string=w376:string)
        n274 = TCP Write(connection ID=w382, data in=w376, error in (no error)=w381) -> (connection ID out=w375:refnum<k5>, error out=w374:errorcluster)  [unwired: 1 in, 1 out]
        n275 = TCP Write(connection ID=w375, data in=w371, error in (no error)=w374) -> (connection ID out=w373:refnum<k5>, error out=w372:errorcluster)  [unwired: 1 in, 1 out]
        n276 = TCP Close Connection(connection ID=w373, error in (no error)=w372) -> ()  [unwired: 1 in, 2 out]
      }
      event "Alarm 5": Value Change {
        w383 = "Alarm Zone 5 "
        n277 = event-data() -> ()  [unwired: 1 in, 6 out]
        n278 = TCP Open Connection(remote port or service name=u16 65529, timeout ms (60000)=60000) -> (connection ID=w394:refnum<k5>, error out=w393:errorcluster)  [unwired: 3 in]
        n279 = String Length(string=w383) -> (length=w390:i32)
        n280 = Number To Decimal String(number=w390, width (-)=i16 1) -> (decimal integer string=w388:string)
        n281 = TCP Write(connection ID=w394, data in=w388, error in (no error)=w393) -> (connection ID out=w387:refnum<k5>, error out=w386:errorcluster)  [unwired: 1 in, 1 out]
        n282 = TCP Write(connection ID=w387, data in=w383, error in (no error)=w386) -> (connection ID out=w385:refnum<k5>, error out=w384:errorcluster)  [unwired: 1 in, 1 out]
        n283 = TCP Close Connection(connection ID=w385, error in (no error)=w384) -> ()  [unwired: 1 in, 2 out]
      }
      event "Alarm 6": Value Change {
        w395 = "Alarm Zone 6 "
        n284 = event-data() -> ()  [unwired: 1 in, 6 out]
        n285 = TCP Open Connection(remote port or service name=u16 65529, timeout ms (60000)=60000) -> (connection ID=w406:refnum<k5>, error out=w405:errorcluster)  [unwired: 3 in]
        n286 = String Length(string=w395) -> (length=w402:i32)
        n287 = Number To Decimal String(number=w402, width (-)=i16 1) -> (decimal integer string=w400:string)
        n288 = TCP Write(connection ID=w406, data in=w400, error in (no error)=w405) -> (connection ID out=w399:refnum<k5>, error out=w398:errorcluster)  [unwired: 1 in, 1 out]
        n289 = TCP Write(connection ID=w399, data in=w395, error in (no error)=w398) -> (connection ID out=w397:refnum<k5>, error out=w396:errorcluster)  [unwired: 1 in, 1 out]
        n290 = TCP Close Connection(connection ID=w397, error in (no error)=w396) -> ()  [unwired: 1 in, 2 out]
      }
    }
  }
